vi "Comp_64_Elements.vi"(10 "Array":u16[](array[numeric])=[0, 0, 0, 0, 0, 0, 0, 0, 0, 0, 0, 0, 0, 0, 0, 0, 0, 0, 0, 0, 0, 0, 0, 0, 0, 0, 0, 0, 0, 0, 0, 0, 0, 0, 0, 0, 0, 0, 0, 0, 0, 0, 0, 0, 0, 0, 0, 0, 0, 0, 0, 0, 0, 0, 0, 0, 0, 0, 0, 0, 0, 0, 0, 0], 11 "CompVal":u16) -> (3 "Boolean":bool)   [LabVIEW 2016]
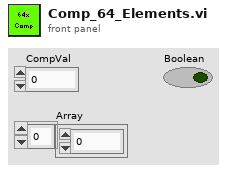
[diagram p1: front panel]
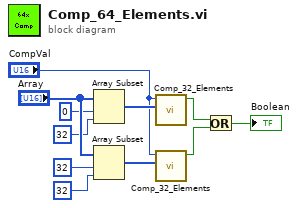
[diagram p0: block diagram]
diagram:
  n1 = Array Subset(array="Array", index=0, length=32 ("index")) -> (w4:u16[])
  n2 = Array Subset(array="Array", index=32, length=32 ("index")) -> (w8:u16[])
  n3 = call "Comp_32_Elements.vi"("Array"=w4, "CompVal"="CompVal") -> ("Result"=w9:bool)  [unwired: 9 in]
  n4 = call "Comp_32_Elements.vi"("Array"=w8, "CompVal"="CompVal") -> ("Result"=w10:bool)  [unwired: 9 in]
  n5 = Or(x=w9, y=w10) -> (x .or. y?=→"Boolean":bool)
